vi "PV_TimeSyncServ_Test.vi"() -> ()   [LabVIEW 2019]
uses:
  <vilib>/Rock Robotics/WPI/ThirdParty/PhotonVisionLib/SubVI/PhotonVision_Globals.vi
  <vilib>/Rock Robotics/WPI/ThirdParty/PhotonVisionLib/PhotonVisionLib.lvlib
panel:
  out "PV_TimeSyncServRcvIP":u32
  out "PV_TimeSyncServReadErr":bool
  out "PV_TimeSyncServWriteErr":bool
  out "PV_TimeSyncLastRcvVer":i8
  out "PV_TimeSyncLoopCount":i32
  out "PV_TimeSyncLastRcvId":i8
  out "PV_TimeSyncLastRcvTim":i64
  out "PV_TimeSyncLastSentTime":i64
  out "PV_TimeSyncStopServ":bool
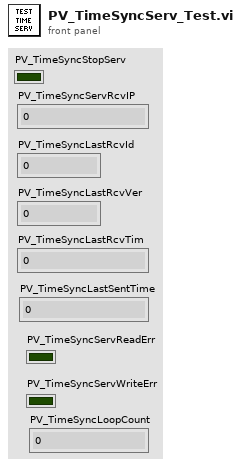
[diagram p1: front panel]
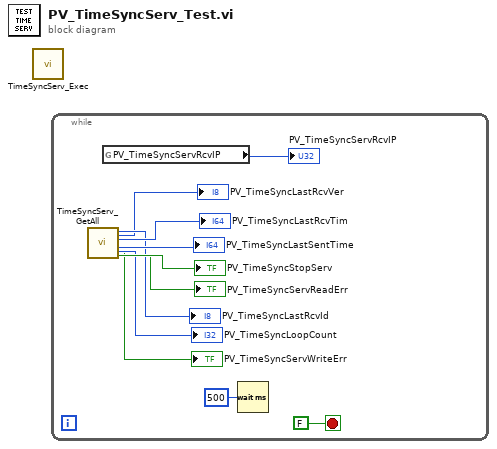
[diagram p0: block diagram]
diagram:
  n1 = call <vilib>:"TimeSyncServ_Exec.vi"() -> ()  [unwired: 12 in]
  n2 = while {
    stop <- FALSE stop-if-true
    n3 = call <vilib>:"TimeSyncServ_GetAll.vi"() -> ("PV_TimeSyncStopServ"=→"PV_TimeSyncStopServ":bool, "PV_TimeSyncLastSentTime"=→"PV_TimeSyncLastSentTime":i64, "PV_TimeSyncLastRcvTim"=→"PV_TimeSyncLastRcvTim":i64, "PV_TimeSyncLastRcvId"=→"PV_TimeSyncLastRcvId":i8, "PV_TimeSyncLoopCount"=→"PV_TimeSyncLoopCount":i32, "PV_TimeSyncLastRcvVer"=→"PV_TimeSyncLastRcvVer":i8, "PV_TimeSyncServWriteErr"=→"PV_TimeSyncServWriteErr":bool, "PV_TimeSyncServReadErr"=→"PV_TimeSyncServReadErr":bool)  [unwired: 3 in, 1 out]
    n4 = global read "PhotonVision_Globals.vi" "PV_TimeSyncServRcvIP"() -> (→"PV_TimeSyncServRcvIP":u32)
    n5 = Wait (ms)(milliseconds to wait=u32 500) -> ()  [unwired: 1 out]
  }
